vi "sub_pkt_parser.vi"(8 "accesscode (bit)":i8[](array[numeric]), 11 "bitstream":i8[](array[numeric])) -> (3 "parsed packet":cluster{"t":u32, "byte_array":u8[]}[](array[cluster]))   [LabVIEW 2014]
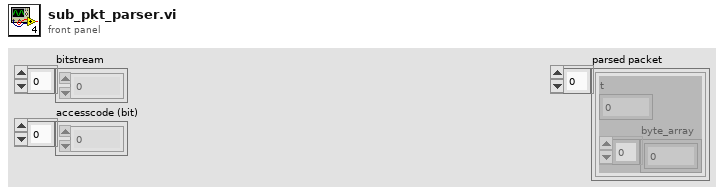
[diagram p1: front panel]
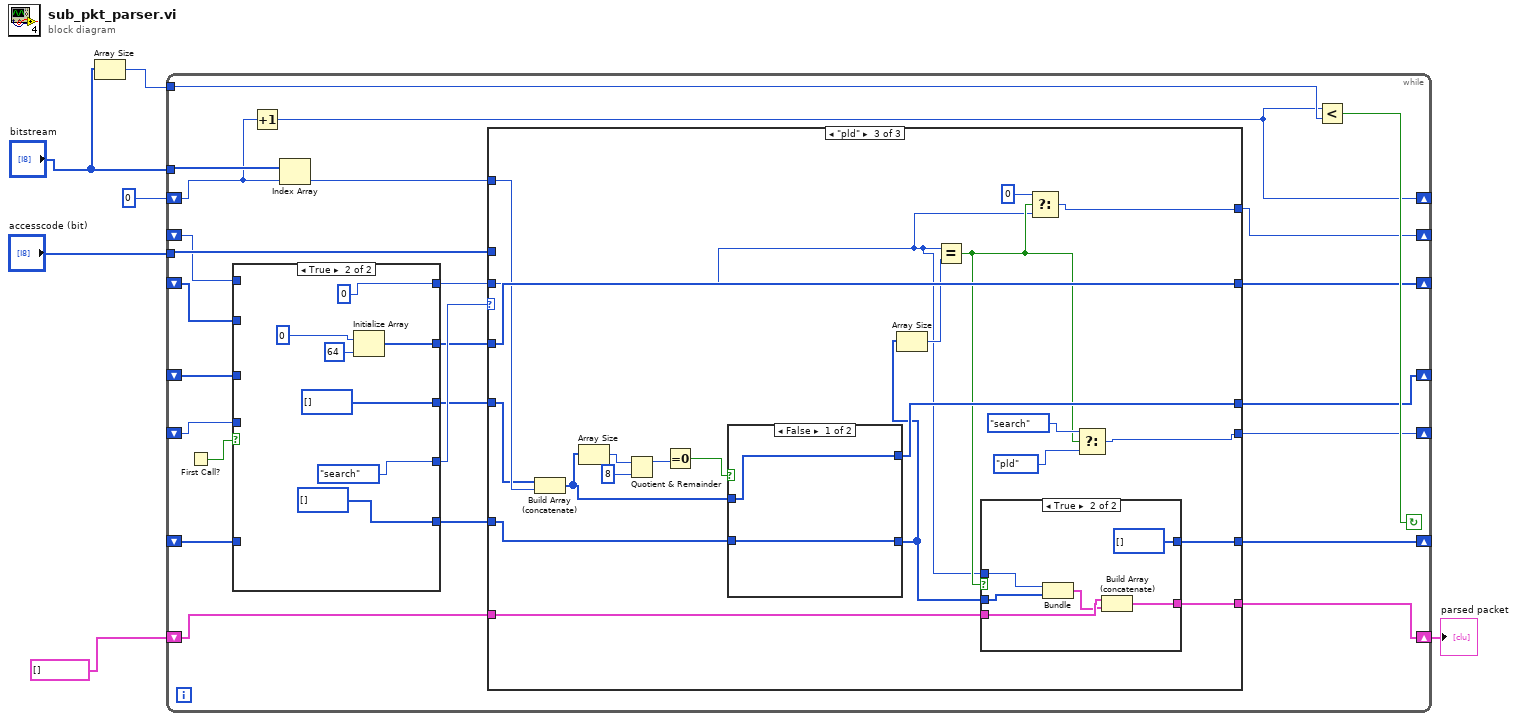
[diagram p0: block diagram]
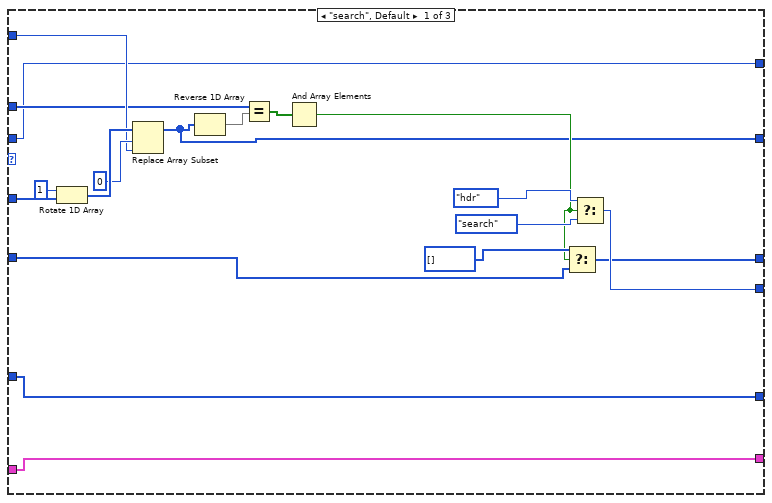
[diagram p2: hidden frame]
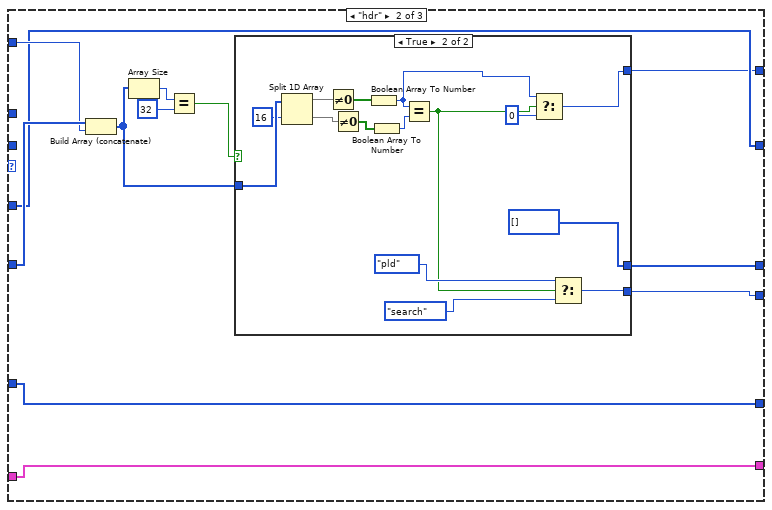
[diagram p3: hidden frame]
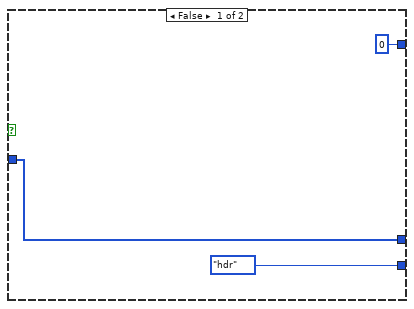
[diagram p4: hidden frame]
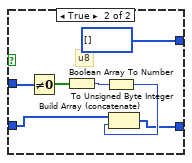
[diagram p6: hidden frame]
diagram:
  n1 = Array Size(array="bitstream") -> (size(s)=w3:i32)
  n2 = while {
    shift-right: [w18] -> _
    shift-left: _ -> [w17]
    tunnel: "bitstream" -> [w29]
    shift-right: [w25] -> _
    shift-left: 0 -> [w28]
    tunnel: "accesscode (bit)" -> [w21]
    tunnel: w3 -> [w27]
    shift-right: [w20] -> _
    shift-left: _ -> [w19]
    shift-right: [w16] -> _
    shift-left: _ -> [w15]
    shift-right: [w13] -> _
    shift-left: _ -> [w12]
    shift-right: [w10] -> _
    shift-left: _ -> [w9]
    shift-right: [w7] -> w1
    shift-left: cluster{"pld_len":u16, "byte_array":u8[]}[] [] -> [w8]
    stop <- w26 continue-if-true
    n3 = First Call?() -> (First Call?: T/F=w31:bool)
    n4 = case shown="True" w31 {
      tunnel: [w123 w129] -> w24
      tunnel: [w122 i8[] []] -> w23
      tunnel: [w124 enum16{"search", "hdr", "pld"}."search"] -> w30
      tunnel: w19 -> [w124 _]
      tunnel: w17 -> [w122 _]
      tunnel: w15 -> [w123 _]
      tunnel: [w121 0] -> w14
      tunnel: w12 -> [w121 _]
      tunnel: [w120 u8[] []] -> w11
      tunnel: w9 -> [w120 _]
      frame False {
      }
      frame True {
        n5 = Initialize Array(i8 0, 64 ("dimension size")) -> (w129:i8[])
      }
    }
    n6 = Increment(x=w28) -> (x+1=w25:i32)
    n7 = Index Array(array=w29, index=w28) -> (element=w22:i8)
    n8 = case shown="\"pld\"" w30 {
      tunnel: w24 -> [w50 w54 w102]
      tunnel: w23 -> [w37 w62 w92]
      tunnel: w22 -> [w46 w61 w98]
      tunnel: w21 -> [w45 _ _]
      tunnel: [w41 w55 w99] -> w20
      tunnel: [w38 w56 w90] -> w18
      tunnel: [w32 w54 w102] -> w16
      tunnel: w14 -> [w33 _ w83]
      tunnel: [w33 w53 w87] -> w13
      tunnel: w11 -> [w34 w51 w91]
      tunnel: [w34 w51 w81] -> w10
      tunnel: w8 -> [w35 w52 w85]
      tunnel: [w35 w52 w82] -> w7
      frame "search", Default {
        n9 = Rotate 1D Array(1:w50, 2:1 ("n")) -> (0:w48:i8[])
        n10 = Replace Array Subset(array=w48, new element=w46, index=0) -> (w32:i8[])
        n11 = Reverse 1D Array(array=w32) -> (reversed array=w36:i8[])
        n12 = Equal?(x=w45, y=w36) -> (x = y?=w44:bool[])
        n13 = And Array Elements(Boolean array=w44) -> (logical AND=w39:bool)
        n14 = Select(t=i8[] [], s=w39, f=w37) -> (s? t:f=w38:i8[])
        n15 = Select(t=enum16{"search", "hdr", "pld"}."hdr", s=w39, f=enum16{"search", "hdr", "pld"}."search") -> (s? t:f=w41:enum16{"search", "hdr", "pld"})
      }
      frame "hdr" {
        n16 = Build Array (concatenate)(w62, w61) -> (w57:i8[])
        n17 = Array Size(array=w57) -> (size(s)=w60:i32)
        n18 = Equal?(x=w60, y=32) -> (x = y?=w58:bool)
        n19 = case shown="True" w58 {
          tunnel: w57 -> [w65 w76]
          tunnel: [w65 i8[] []] -> w56
          tunnel: [enum16{"search", "hdr", "pld"}."hdr" w80] -> w55
          tunnel: [u32 0 ("f") w67] -> w53
          frame False {
          }
          frame True {
            n20 = Split 1D Array(array=w76, index=16) -> (first subarray=w74:i8[], second subarray=w73:i8[])
            n21 = Not Equal To 0?(x=w74) -> (x != 0?=w72:bool[])
            n22 = Not Equal To 0?(x=w73) -> (x != 0?=w71:bool[])
            n23 = Boolean Array To Number(Boolean array=w72) -> (number=w66:u32)
            n24 = Boolean Array To Number(Boolean array=w71) -> (number=w70:u32)
            n25 = Equal?(x=w66, y=w70) -> (x = y?=w69:bool)
            n26 = Select(t=w66, s=w69, f=0) -> (s? t:f=w67:u32)
            n27 = Select(t=enum16{"search", "hdr", "pld"}."pld", s=w69, f=enum16{"search", "hdr", "pld"}."search") -> (s? t:f=w80:enum16{"search", "hdr", "pld"})
          }
        }
      }
      frame "pld" {
        n28 = Build Array (concatenate)(w92, w98) -> (w93:i8[])
        n29 = Array Size(array=w93) -> (size(s)=w97:i32)
        n30 = Quotient & Remainder(x=w97, y=8) -> (x-y*floor(x/y)=w95:i32)  [unwired: 1 out]
        n31 = Equal To 0?(x=w95) -> (x = 0?=w94:bool)
        n32 = case shown="False" w94 {
          tunnel: w93 -> [w112 w119]
          tunnel: w91 -> [w111 w117]
          tunnel: [w111 w114] -> w84
          tunnel: [w112 i8[] []] -> w90
          frame False {
          }
          frame True {
            # "u8"
            n33 = Not Equal To 0?(x=w119) -> (x != 0?=w118:bool[])
            n34 = Boolean Array To Number(Boolean array=w118) -> (number=w116:u32)
            n35 = To Unsigned Byte Integer(number=w116) -> (unsigned 8bit integer=w115:u8)
            n36 = Build Array (concatenate)(w117, w115) -> (w114:u8[])
          }
        }
        n37 = Array Size(array=w84) -> (size(s)=w89:i32)
        n38 = Equal?(x=w83, y=w89) -> (x = y?=w86:bool)
        n39 = case shown="True" w86 {
          tunnel: w85 -> [w103 w108]
          tunnel: w84 -> [w104 w110]
          tunnel: w83 -> [_ w109]
          tunnel: [w103 w106] -> w82
          tunnel: [w104 u8[] []] -> w81
          frame False {
          }
          frame True {
            n40 = Bundle("t"=w109, w110) -> (w107:cluster{"t":u32, u8[]})  [unwired: 1 in]
            n41 = Build Array (concatenate)(w108, w107) -> (w106:cluster{"t":u32, "byte_array":u8[]}[])
          }
        }
        n42 = Select(t=u32 0, s=w86, f=w83) -> (s? t:f=w87:u32)
        n43 = Select(t=enum16{"search", "hdr", "pld"}."search", s=w86, f=enum16{"search", "hdr", "pld"}."pld") -> (s? t:f=w99:enum16{"search", "hdr", "pld"})
      }
    }
    n44 = Less?(x=w25, y=w27) -> (x < y?=w26:bool)
  }
  "parsed packet" <- w1
